vi "CycleRemoveGroup.vi"(11 "TreeControl输入":refnum<vi>) -> (0 "删除的行数":i32, 1 "删除起始行索引":i32, 3 "TreeControl输出":refnum<vi>)   [LabVIEW 2020, in "Curve Editor.lvlib"]
uses:
  Curve Editor.lvlib
panel:
  # "删除树形中选中的组标识及其子标识，并返回删除起始的行索引及删除掉的行数"
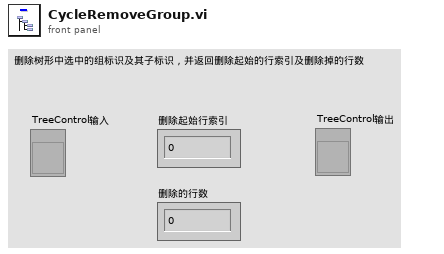
[diagram p1: front panel]
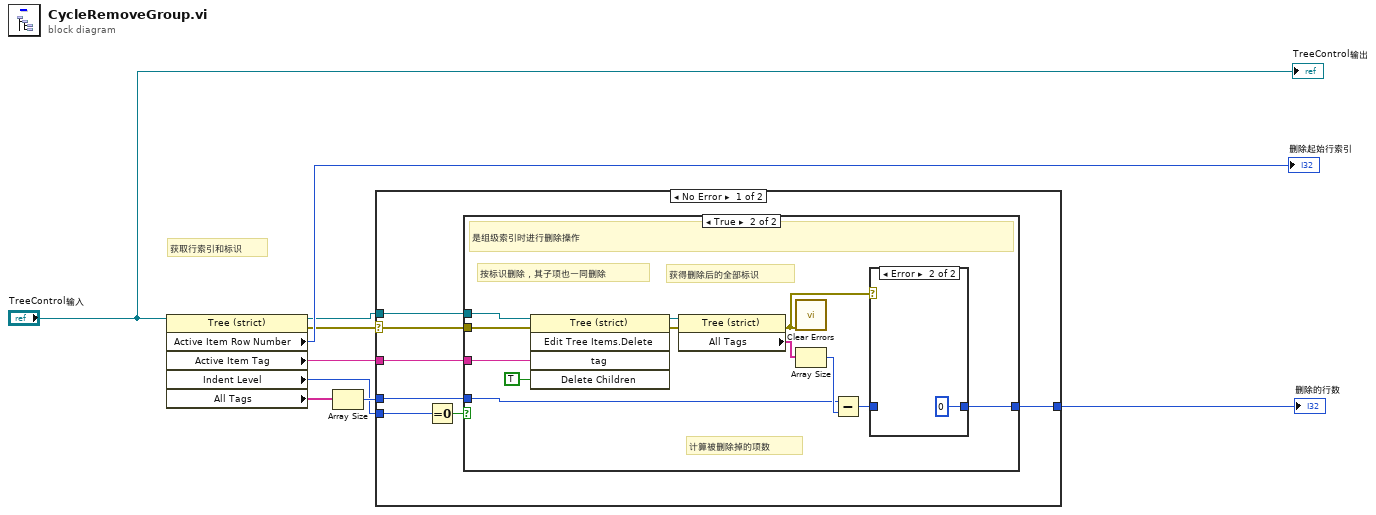
[diagram p0: block diagram]
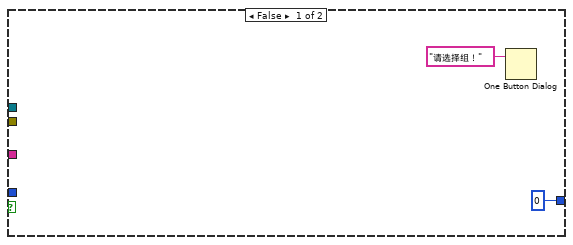
[diagram p2: hidden frame]
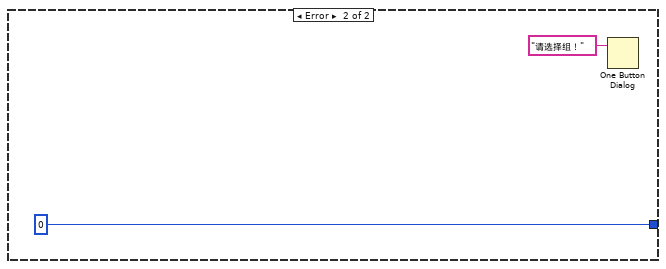
[diagram p4: hidden frame]
diagram:
  # "获取行索引和标识"
  n1 = property class="Tree (strict)"(reference="TreeControl输入") -> (reference out=w4:refnum<vi>, error out=w5:errorcluster, "Active Item Row Number"=→"删除起始行索引":i32, "Active Item Tag"=w3:string, "Indent Level"=w2:i32, "All Tags"=w7:string[])  [unwired: 1 in]
  n2 = Array Size(array=w7) -> (size(s)=w8:i32)
  n3 = case shown="No Error" w5 {
    selector: w5 -> [w13 _]
    tunnel: w2 -> [w16 _]
    tunnel: w3 -> [w15 _]
    tunnel: w4 -> [w10 _]
    tunnel: w8 -> [w12 _]
    tunnel: [w11 0] -> w9
    frame No Error {
      n4 = Equal To 0?(x=w16) -> (x = 0?=w14:bool)
      n5 = case shown="True" w14 {
        tunnel: w15 -> [_ w30]
        tunnel: w10 -> [_ w28]
        tunnel: w13 -> [_ w27]
        tunnel: w12 -> [_ w22]
        tunnel: [0 w19] -> w11
        frame False {
          n6 = One Button Dialog(message="请选择组！" ("消息")) -> ()  [unwired: 1 in, 1 out]
        }
        frame True {
          # "计算被删除掉的项数"
          # "获得删除后的全部标识"
          # "按标识删除，其子项也一同删除"
          # "是组级索引时进行删除操作"
          n7 = invoke class="Tree (strict)" method="Edit Tree Items.Delete"(reference=w28, error in=w27, "tag"=w30, "Delete Children"=TRUE ("删除子项？")) -> (reference out=w26:refnum<vi>, error out=w25:errorcluster)  [unwired: 1 in, 3 out]
          n8 = property class="Tree (strict)"(reference=w26, error in=w25) -> (error out=w21:errorcluster, "All Tags"=w24:string[])  [unwired: 1 out]
          n9 = call <vilib>:"Clear Errors.vi"("error in (no error)"=w21) -> ()  [unwired: 5 in, 2 out]
          n10 = Array Size(array=w24) -> (size(s)=w23:i32)
          n11 = Subtract(x=w22, y=w23) -> (x-y=w20:i32)
          n12 = case shown="Error" w21 {
            tunnel: w20 -> [w31 _]
            tunnel: [w31 0] -> w19
            frame No Error {
            }
            frame Error {
            }
          }
        }
      }
    }
    frame Error {
      n13 = One Button Dialog(message="请选择组！" ("消息")) -> ()  [unwired: 1 in, 1 out]
    }
  }
  "删除的行数" <- w9
  "TreeControl输出" <- "TreeControl输入"
